vi "Clear.vi"(8 "error in (no error)":errorcluster, 11 "Base In":refnum<class "Base.lvclass">) -> (0 "error out":errorcluster, 3 "Base Out":refnum<class "Base.lvclass">)   [LabVIEW 2020, in "Base.lvclass"]
doc: "Clears any resorces allocated during initialization."
uses:
  Base.lvclass
  Base.lvclass/Base.ctl
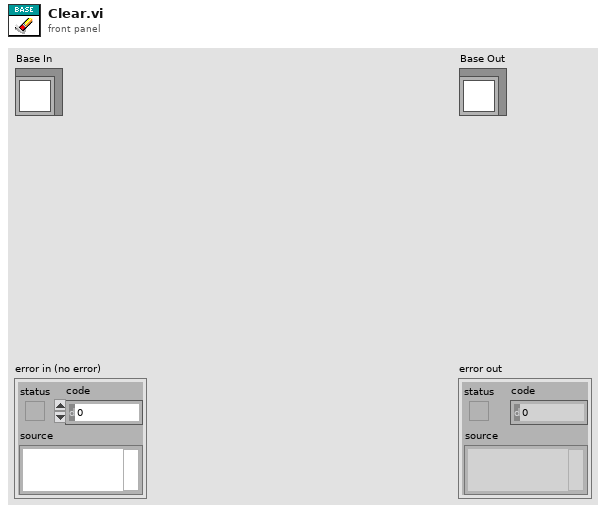
[diagram p1: front panel]
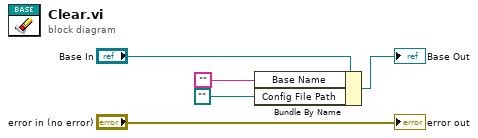
[diagram p0: block diagram]
diagram:
  n1 = Bundle By Name(cluster="Base In", "Base Name"="", "Config File Path"=path "") -> (→"Base Out":refnum<class "Base.lvclass">)
  "error out" <- "error in (no error)"
